vi "Save Cursors.vi"(8 "error in (no error)":errorcluster, 11 "Cursor List":T1) -> (0 "error out":errorcluster, 3 "Cursor List 2":T1)   [LabVIEW 2014, in "Map Data.lvlib"]
doc: "Updates an existing contact or inserts a new contact into the address book data store. Use the ID of an existing contact to update, or an ID of 0 to insert. When inserting, the output cluster will contain the ID of the new contact."
uses:
  Map Data.lvlib
  CursorList.ctl
  MapCommand.ctl
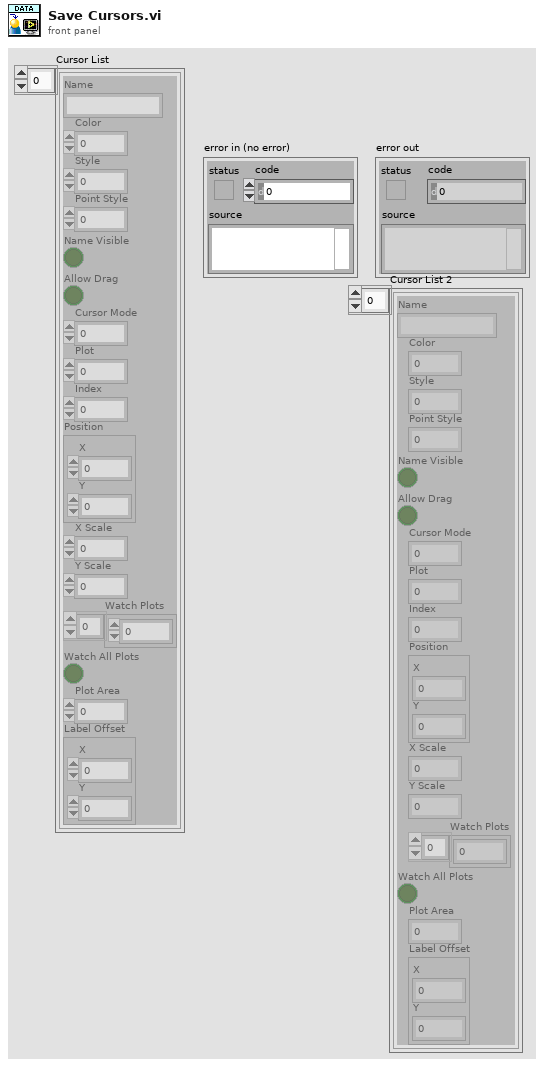
[diagram p1: front panel]
types:
  T1 = typedef "Map Data.lvlib/CursorList.ctl" = cluster{"Name":string, "Color":u32, "Style":u8, "Point Style":u8, "Name Visible":bool, "Allow Drag":bool, "Cursor Mode":u32, "Plot":i32, "Index":i32, "Position":cluster{"X":dbl, "Y":dbl}, "X Scale":u32, "Y Scale":u32, "Watch Plots":i32[], "Watch All Plots":bool, "Plot Area":i32, "Label Offset":cluster{"X":dbl, "Y":dbl}}[]
  T2 = typedef "Map Data.lvlib/MapCommand.ctl" = enum16{"Load", "Update Cursor", "Save", "Get All Data", "Get Single Data", "Set Single Data", "Delete All", "Remove Single Data", "Set Favorite Status", "Is Data Modified", "Import Data"}
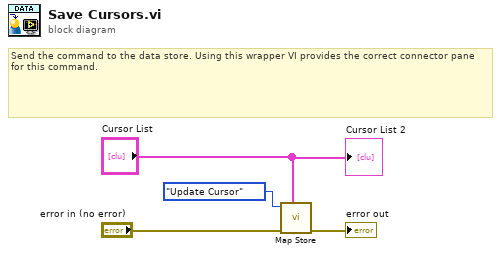
[diagram p0: block diagram]
diagram:
  # "Send the command to the data store. Using this wrapper VI provides the correct connector pane for this command."
  n1 = call "Map Store.vi"("Cursor List"="Cursor List", "error in (no error)"="error in (no error)", "Command"=MapCommand."Update Cursor") -> ("error out"=→"error out":errorcluster)  [unwired: 5 in, 3 out]
  "Cursor List 2" <- "Cursor List"
